vi "Custom waveform signal generation.vi"() -> ()   [LabVIEW 2010]
doc: "This example shows how to program Red Pitaya to generate custom waveform signal. Red Pitaya is able to generate signals in range from DC to 50 MHz with output voltage range from -1 to 1 Volt. Generated signal can be observed by Red Pitaya Oscilloscope WEB application. To run it, just open web browser, input Red Pitaya IP and start Oscilloscope."
uses:
  RedPitaya.lvlib
panel:
  in  "file path (dialog if empty)":path
  out "Waveform Graph 2":dbl[](graph)
  out "Waveform Graph 1":dbl[](graph)
  in  "IP address":string="192.168.1.100"
  # "If you leave file path empty,\narbitrary waveform on Ch2\nwill be generated using for loop.\nIf you set file path to CSV file,\narbitrary waveform on Ch2\nwill be generated using data in\nCSV file."
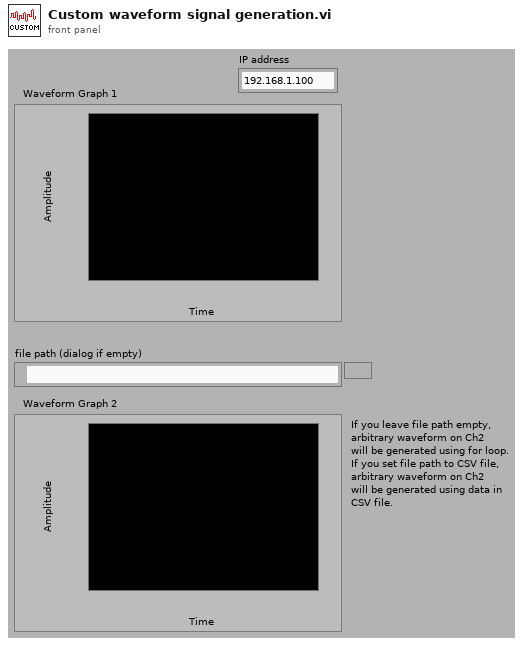
[diagram p1: front panel]
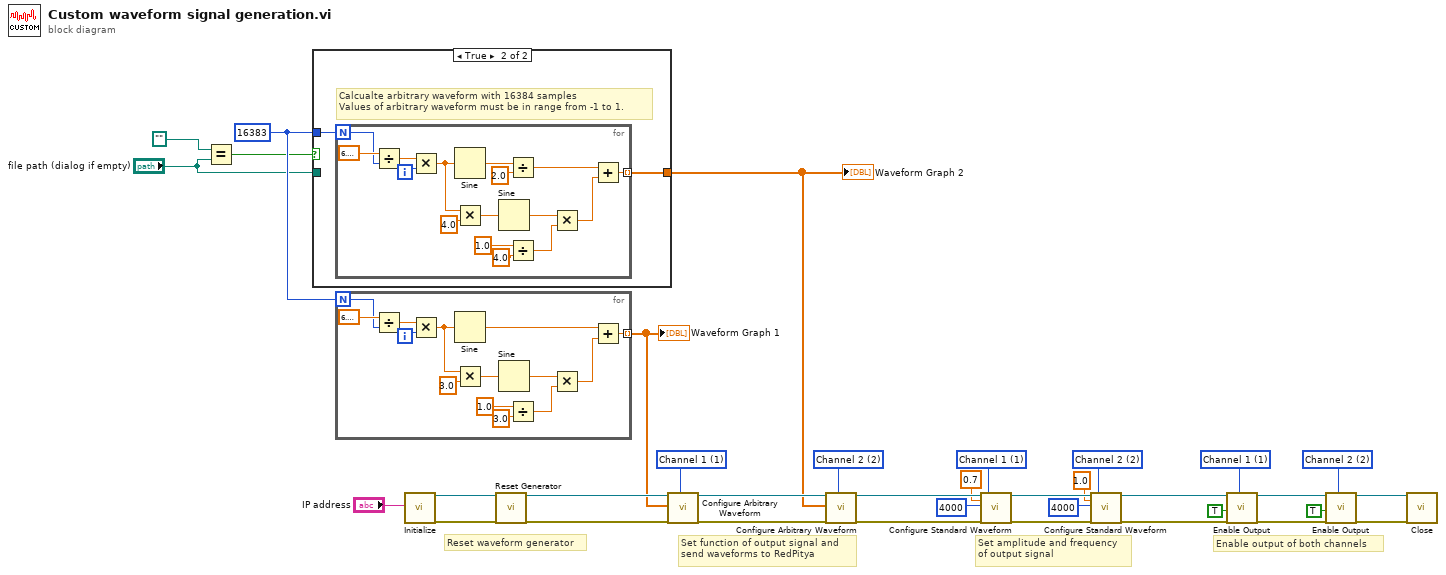
[diagram p0: block diagram]
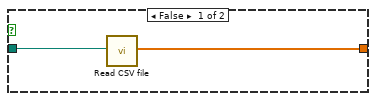
[diagram p2: hidden frame]
diagram:
  w10 = u16 2 items=["Channel 1"=1, "Channel 2"=2] ("Channel #")
  w20 = u16 2 items=["Channel 1"=1, "Channel 2"=2] ("Channel (1|2)")
  w21 = u16 1 items=["Channel 1"=1, "Channel 2"=2] ("Channel (1|2)")
  w8 = 2 items=["Channel 1"=1, "Channel 2"=2] ("Channel (0: 1)")
  w33 = 16383
  w9 = 1 items=["Channel 1"=1, "Channel 2"=2] ("Channel (0: 1)")
  w7 = u16 1 items=["Channel 1"=1, "Channel 2"=2] ("Channel (1|2)")
  # "Reset waveform generator"
  # "Enable output of both channels"
  # "Set amplitude and frequency\nof output signal"
  # "Set function of output signal and\nsend waveforms to RedPitya"
  n1 = Equal?(x=path "", y="file path (dialog if empty)") -> (x = y?=w2:bool)
  n2 = case shown="True" w2 {
    tunnel: w33 -> [_ w39]
    tunnel: [w36 w38] -> w12
    tunnel: "file path (dialog if empty)" -> [w37 _]
    frame False {
      n3 = call "Read CSV file.vi"("file path (dialog if empty)"=w37) -> ("row"=w36:dbl[])  [unwired: 18 in]
    }
    frame True {
      # "Calcualte arbitrary waveform with 16384 samples\nValues of arbitrary waveform must be in range from -1 to 1."
      n4 = for {
        N: w39 -> [w46]
        tunnel: [w47] -> w38 mode=indexing
        i -> [w44]
        n5 = Divide(x=6.283185307179586, y=w46) -> (x/y=w45:dbl)
        n6 = Multiply(x=w45, y=w44) -> (x*y=w43:dbl)
        n7 = Sine(x=w43) -> (sin(x)=w42:dbl)
        n8 = Multiply(x=w43, y=4.0) -> (x*y=w53:dbl)
        n9 = Sine(x=w53) -> (sin(x)=w50:dbl)
        n10 = Divide(x=w42, y=2.0) -> (x/y=w40:dbl)
        n11 = Divide(x=1.0, y=4.0) -> (x/y=w49:dbl)
        n12 = Multiply(x=w50, y=w49) -> (x*y=w48:dbl)
        n13 = Add(x=w40, y=w48) -> (x+y=w47:dbl)
      }
    }
  }
  "Waveform Graph 2" <- w12
  n14 = for {
    N: w33 -> [w59]
    tunnel: [w60] -> w11 mode=indexing
    i -> [w57]
    n15 = Divide(x=6.283185307179586, y=w59) -> (x/y=w58:dbl)
    n16 = Multiply(x=w58, y=w57) -> (x*y=w56:dbl)
    n17 = Sine(x=w56) -> (sin(x)=w62:dbl)
    n18 = Multiply(x=w56, y=3.0) -> (x*y=w67:dbl)
    n19 = Sine(x=w67) -> (sin(x)=w64:dbl)
    n20 = Divide(x=1.0, y=3.0) -> (x/y=w63:dbl)
    n21 = Multiply(x=w64, y=w63) -> (x*y=w61:dbl)
    n22 = Add(x=w62, y=w61) -> (x+y=w60:dbl)
  }
  "Waveform Graph 1" <- w11
  n23 = call "Initialize.vi"("IP address"="IP address") -> ("RedPitaya connection out"=w15:refnum<k5>, "error out"=w13:errorcluster)  [unwired: 17 in]
  n24 = call "Reset Generator.vi"("RedPitaya connection in"=w15, "error in"=w13) -> ("RedPitaya connection out"=w14:refnum<k5>, "error out"=w6:errorcluster)  [unwired: 16 in]
  n25 = call "Configure Arbitrary Waveform.vi"("RedPitaya connection in"=w14, "Data"=w11, "error in"=w6, "Channel #"=w7) -> ("RedPitaya connection out"=w32:refnum<k5>, "error out"=w5:errorcluster)  [unwired: 14 in]
  n26 = call "Configure Arbitrary Waveform.vi"("RedPitaya connection in"=w32, "Data"=w12, "error in"=w5, "Channel #"=w10) -> ("RedPitaya connection out"=w26:refnum<k5>, "error out"=w4:errorcluster)  [unwired: 14 in]
  n27 = call "Configure Standard Waveform.vi"("RedPitaya connection in"=w26, "Amplitude (V)"=0.7 ("Amplitude"), "Frequency"=4000 ("Frequency (1000 Hz)"), "error in"=w4, "Channel #"=w21) -> ("RedPitaya connection out"=w25:refnum<k5>, "error out"=w22:errorcluster)  [unwired: 13 in]
  n28 = call "Configure Standard Waveform.vi"("RedPitaya connection in"=w25, "Amplitude (V)"=1.0 ("Amplitude"), "Frequency"=4000 ("Frequency (1000 Hz)"), "error in"=w22, "Channel #"=w20) -> ("RedPitaya connection out"=w24:refnum<k5>, "error out"=w23:errorcluster)  [unwired: 13 in]
  n29 = call "Enable Output.vi"("RedPitaya connection in"=w24, "Generation (T: Enable)"=TRUE, "error in"=w23, "Channel #"=w9) -> ("RedPitaya connection out"=w31:refnum<k5>, "error out"=w30:errorcluster)  [unwired: 14 in]
  n30 = call "Enable Output.vi"("RedPitaya connection in"=w31, "Generation (T: Enable)"=TRUE, "error in"=w30, "Channel #"=w8) -> ("RedPitaya connection out"=w28:refnum<k5>, "error out"=w27:errorcluster)  [unwired: 14 in]
  n31 = call "Close.vi"("RedPitaya connection in"=w28, "error in"=w27) -> ()  [unwired: 17 in, 1 out]
